vi "CSMP-Broadcast.vi"(0 "state":string, 1 "args":string, 2 "source/target":string, 5 "Error in":errorcluster caption="Error in (no error)", 8 "Module Name":string, 10 "Msg Type":T1=enum."Broadcast(-><status>)") -> (14 "state out":string, 15 "args out":string, 16 "source/target out":string, 17 "Pre-State out":string, 18 "Pre-Args out":string, 19 "error":errorcluster)   [LabVIEW 2020, in "Communicable State Machine.lvlib"]
uses:
  Communicable State Machine.lvlib
  _CSM_MSG_TYPE.ctl
  _Cross CSM State Data.ctl
  _Cross CSM State Response.ctl
  _CSM_Response Source Message.ctl
  Priority Queue.lvclass/Priority Queue.ctl
  CSM - Make String Arguments Safe.vi
  Enqueue Element.vi
  Trim Both Whitespace.vi
  CSM - Keywords.vi
  global-CSMQ FGV Change Flag.vi
  global-Broadcast Cache Change Flag.vi
  Broadcast Item Key.vi
  _CSMOFGV.vi
  FGV-BroadcastRegistry.vi
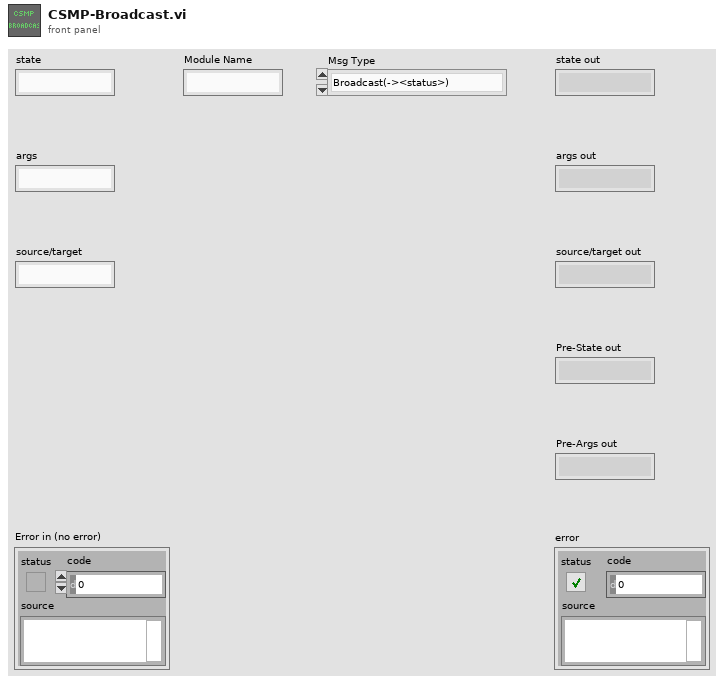
[diagram p1: front panel]
types:
  T1 = typedef "Communicable State Machine.lvlib/_CSM_MSG_TYPE.ctl" = enum16{"Sync Message(-@)", "Async Message(->)", "Async without Response(->|)", "Async Response", "Broadcast(-><all>)", "Broadcast(-><status>)", "Broadcast(-><interrupt>)", "Append to JKISM States", "Append to JKISM States(High Priority)"}
  T2 = typedef "Communicable State Machine.lvlib/CSM - Broadcast Message Type.ctl" = enum16{"Status", "Interrupt(High)"}
  T3 = cluster{"Target CSM":string, "Target State":string, "Priority":T2}[]
  T4 = typedef "Communicable State Machine.lvlib/_Cross CSM State Data.ctl" = cluster{"Msg Type":T1, "state":string, "args":string, "source":string, "RespQ":refnum<queue>, "Response For Message":T5, "Target":string}
  T5 = typedef "Communicable State Machine.lvlib/_CSM_Response Source Message.ctl" = cluster{"‘State":string, "’Arguments":string, "’Error":errorcluster}
  T6 = typedef "Communicable State Machine.lvlib/_CSMObj.ctl" = cluster{"Requested Name":string, "Module Name":string, "Mode":T7, "Queue":refnum<class "Priority Queue.lvclass">, "CSM-Data":refnum<data-value>, "User Event":refnum<user-event>, "Status Change Event":refnum<user-event>, "Allowed Messages":string[], "Mode-Data":refnum<data-value>, "Group Name":string, "Exit Event":refnum<user-event>}
  T7 = typedef "Communicable State Machine.lvlib/_CSM_MODE.ctl" = enum16{"Not Exist", "Stand Alone", "CSM", "Worker Agent", "Worker", "Chain", "Chain Node"}
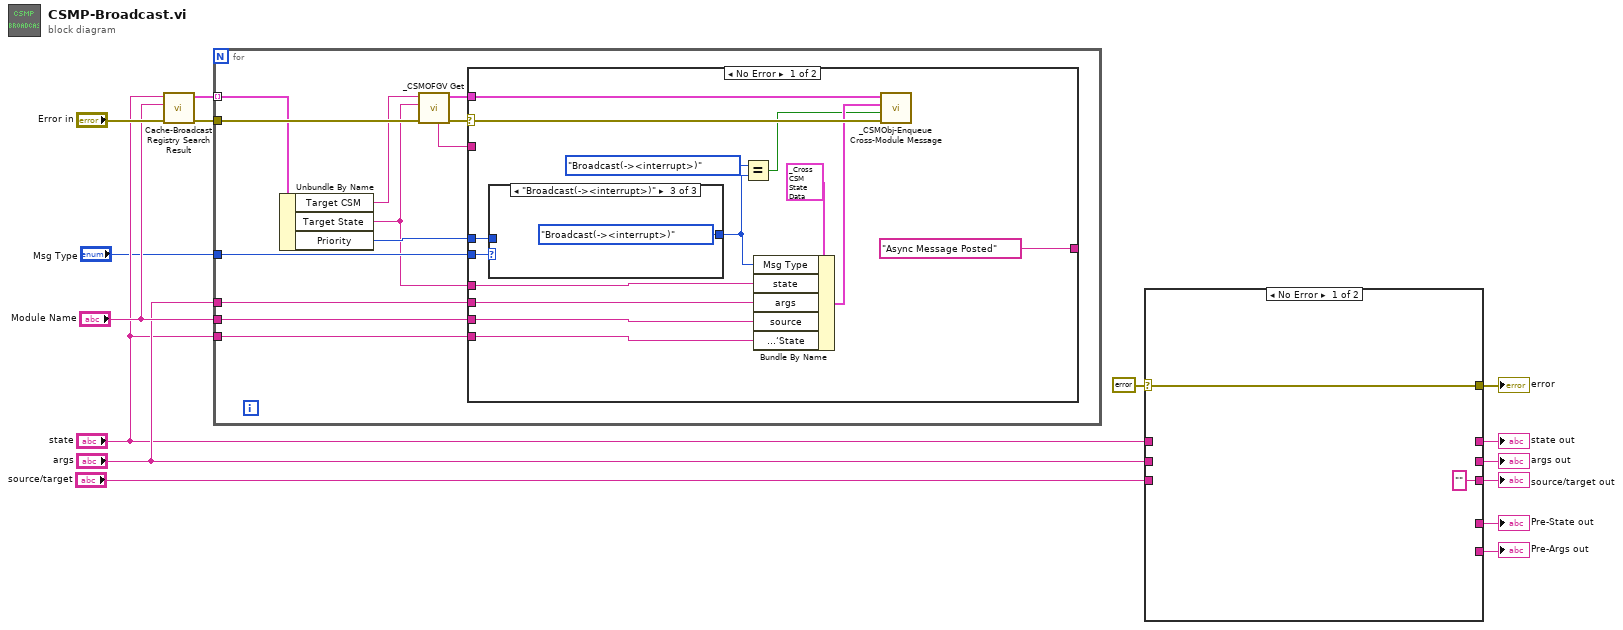
[diagram p0: block diagram]
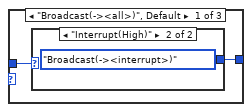
[diagram p2: hidden frame]
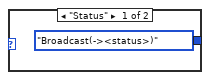
[diagram p3: hidden frame]
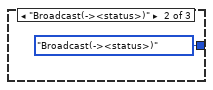
[diagram p4: hidden frame]
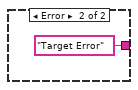
[diagram p5: hidden frame]
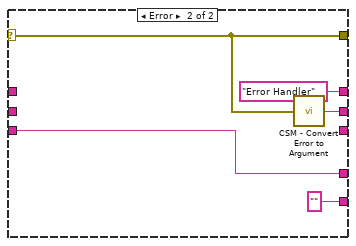
[diagram p6: hidden frame]
diagram:
  n1 = call "Cache-Broadcast Registry Search Result.vi"("error in (no error)"="Error in", "CSM Name"="Module Name", "Broadcast state"="state") -> ("error out"=w8:errorcluster, "Array"=w7:T3)  [unwired: 7 in]
  n2 = for {
    tunnel: w8 -> [w24]
    tunnel: w7 -> [w20] mode=indexing
    tunnel: "args" -> [w23]
    tunnel: "Module Name" -> [w22]
    tunnel: "state" -> [w21]
    tunnel: "Msg Type" -> [w18]
    n3 = Unbundle By Name(w20) -> ("Target CSM"=w19:string, "Target State"=w16:string, "Priority"=w17:T2)
    n4 = call "_CSMOFGV Get.vi"("Error in"=w24, "Message"=w16, "Name(\"\" to use uuid) in"=w19) -> ("Error out"=w26:errorcluster, "CSM-Obj"=w27:T6, "Name"=w25:string)  [unwired: 6 in]
    n5 = case shown="No Error" w26 {
      selector: w26 -> [w40 _]
      tunnel: w27 -> [w41 _]
      tunnel: ["Async Message Posted" ("before match") "Target Error" ("before match")] -> _
      tunnel: w16 -> [w35 _]
      tunnel: w23 -> [w38 _]
      tunnel: w22 -> [w37 _]
      tunnel: w25 -> [_ _]
      tunnel: w21 -> [w34 _]
      tunnel: w18 -> [w29 _]
      tunnel: w17 -> [w31 _]
      frame No Error {
        n6 = case shown="\"Broadcast(-><interrupt>)\"" w29 {
          tunnel: w31 -> [w43 _ _]
          tunnel: [w42 _CSM_MSG_TYPE."Broadcast(-><status>)" ("Msg Type") _CSM_MSG_TYPE."Broadcast(-><interrupt>)" ("Msg Type")] -> w30
          frame "Broadcast(-><all>)", Default {
            n7 = case shown="\"Interrupt(High)\"" w43 {
              tunnel: [_CSM_MSG_TYPE."Broadcast(-><status>)" ("Msg Type") _CSM_MSG_TYPE."Broadcast(-><interrupt>)" ("Msg Type")] -> w42
              frame "Status" {
              }
              frame "Interrupt(High)" {
              }
            }
          }
          frame "Broadcast(-><status>)" {
          }
          frame "Broadcast(-><interrupt>)" {
          }
        }
        n8 = Equal?(x=_CSM_MSG_TYPE."Broadcast(-><interrupt>)", y=w30) -> (x = y?=w32:bool)
        n9 = Bundle By Name(cluster=T4 {"Msg Type"=enum."Sync Message(-@)", "state"="", "args"="", "source"="", "RespQ"=refnum, "Response For Message"={"‘State"="", "’Arguments"="", "’Error"={"status"=FALSE, "code"=0, "source"=""}}, "Target"=""} ("Cross JKI State Machine State"), "Msg Type"=w30, "state"=w35, "args"=w38, "source"=w37, "Response For Message.‘State"=w34) -> (w36:T4)
        n10 = call "_CSMObj-Enqueue Cross-Module Message.vi"("Error in"=w40, "High Priority?(F)"=w32, "Data"=w36, "CSMQ in"=w41) -> ()  [unwired: 6 in, 2 out]
      }
      frame Error {
      }
    }
  }
  n11 = case shown="No Error" errorcluster {"status"=FALSE, "code"=0, "source"=""} ("error IO") {
    selector: errorcluster {"status"=FALSE, "code"=0, "source"=""} ("error IO") -> [w50 w53]
    tunnel: [_ w51] -> w15
    tunnel: [w50 w53] -> w14
    tunnel: [_ "" ("Pre-State out")] -> w13
    tunnel: "state" -> [_ _]
    tunnel: [_ "Error Handler" ("state")] -> w12
    tunnel: "args" -> [_ _]
    tunnel: [_ w52] -> w11
    tunnel: "source/target" -> [_ w51]
    tunnel: ["" ("source/target") _] -> w9
    frame No Error {
    }
    frame Error {
      n12 = call "CSM - Convert Error to Argument.vi"("error in (no error)"=w53) -> ("Arguments"=w52:string)  [unwired: 4 in]
    }
  }
  "state out" <- w12
  "args out" <- w11
  "source/target out" <- w9
  "Pre-State out" <- w15
  "Pre-Args out" <- w13
  "error" <- w14
